vi "Close.vi"(8 "error in (no error)":errorcluster, 11 "eLab in":refnum<class "PL eLabFTW Client.lvclass">) -> (0 "error out":errorcluster)   [LabVIEW 2015, in "PL eLabFTW Client.lvclass"]
doc: "Closes connection to eLabFTW server."
uses:
  PL eLabFTW Client.lvclass
  PL eLabFTW Client.lvclass/PL eLabFTW Client.ctl
  <vilib>/httpClient/LabVIEWHTTPClient.lvlib
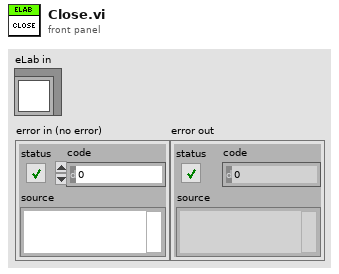
[diagram p1: front panel]
types:
  T1 = typedef "LabVIEWHTTPClient.lvlib/ClientHandle.ctl" = refnum<k1>
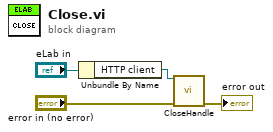
[diagram p0: block diagram]
diagram:
  n1 = Unbundle By Name("eLab in") -> ("HTTP client"=w3:T1)
  n2 = call <vilib>:"CloseHandle.vi"("client handle"=w3, "error in (no error)"="error in (no error)") -> ("error out"=→"error out":errorcluster)  [unwired: 13 in]
